vi "PDE_Fill_Setup(SubVI).vi"(6 "sample mode":i32, 8 "Error In":errorcluster, 9 "rate":dbl, 10 "number of samples":i32, 11 "Input Boolean Array":digitalwaveform[](array[waveform])) -> (0 "error out":errorcluster, 3 "Refnum out":refnum<k21>)   [LabVIEW 2018]
uses:
  <vilib>/DAQmx/write.llb/DAQmx Write (Digital 1D Wfm NChan NSamp).vi
  <vilib>/DAQmx/create/channels.llb/DAQmx Create Channel (DO-Digital Output).vi
  <vilib>/DAQmx/configure/timing.llb/DAQmx Timing (Sample Clock).vi
  <vilib>/Waveform/DWDTOps.llb/DWDT Uncompress Digital.vi
  <vilib>/DAQmx/miscellaneous.llb/DAQmx Fill In Error Info.vi
  <resource>/objmgr/daqmx.rc
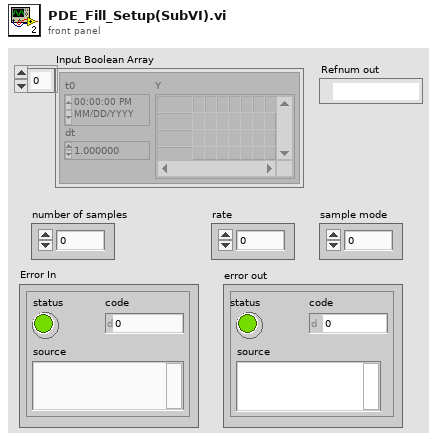
[diagram p1: front panel]
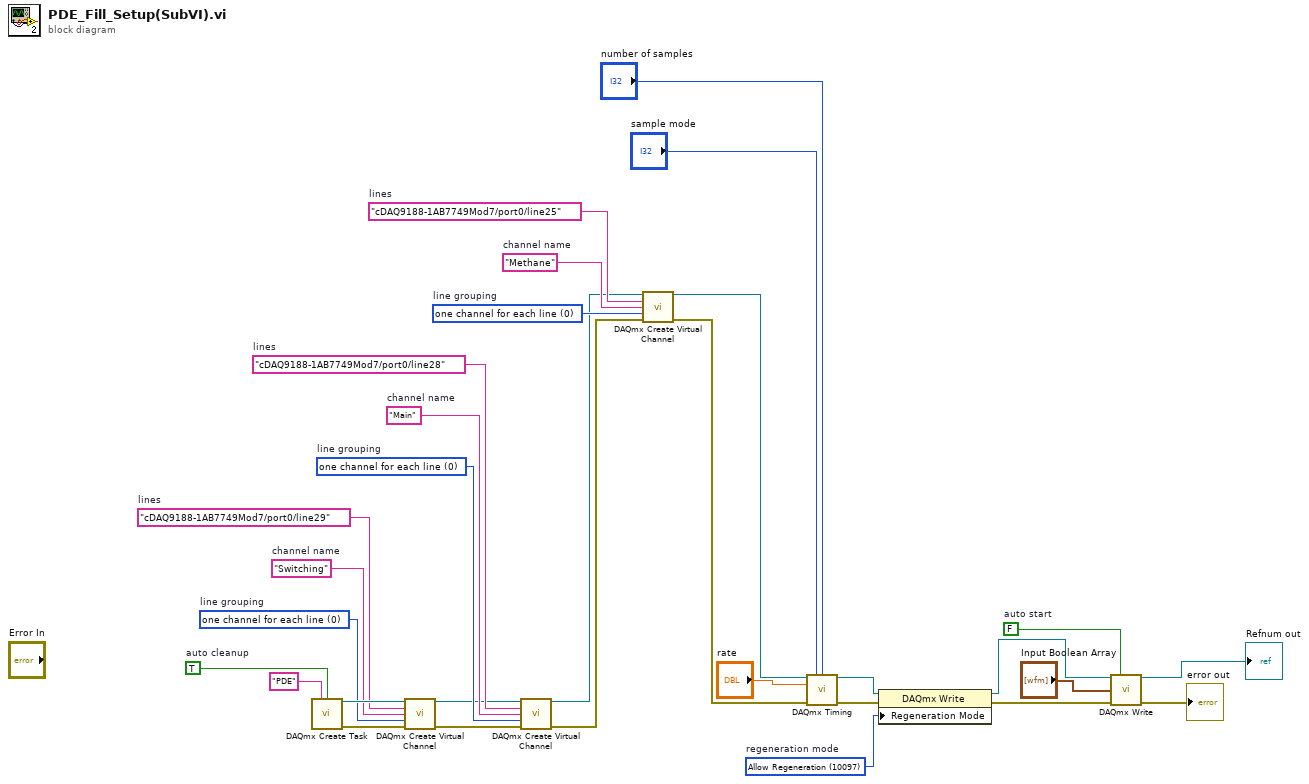
[diagram p0: block diagram]
diagram:
  w21 = 0 items=["one channel for each line", "one channel for all lines"]  # line grouping
  w22 = "Methane"  # channel name
  w20 = "cDAQ9188-1AB7749Mod7/port0/line25"  # lines
  w16 = 0 items=["one channel for each line", "one channel for all lines"]  # line grouping
  w17 = "Main"  # channel name
  w15 = "cDAQ9188-1AB7749Mod7/port0/line28"  # lines
  w11 = 0 items=["one channel for each line", "one channel for all lines"]  # line grouping
  w12 = "Switching"  # channel name
  w10 = "cDAQ9188-1AB7749Mod7/port0/line29"  # lines
  w6 = 10097 items=["Allow Regeneration"=10097, "Do Not Allow Regeneration"=10158]  # regeneration mode
  w3 = TRUE  # auto cleanup
  w1 = FALSE  # auto start
  n1 = call <vilib>:"DAQmx Create Task.vi"("new task name"="PDE", "auto cleanup"=w3) -> ("task out"=w26:refnum<k21>, "error out"=w25:errorcluster)  [unwired: 12 in]
  n2 = call-poly <vilib>:"DAQmx Create Virtual Channel.vi"("task in"=w26, "lines"=w10, "name to assign"=w12, "line grouping"=w11, "error in"=w25) -> ("task out"=w14:refnum<k21>, "error out"=w13:errorcluster)  [unwired: 9 in]
  n3 = call-poly <vilib>:"DAQmx Create Virtual Channel.vi"("task in"=w14, "lines"=w15, "name to assign"=w17, "line grouping"=w16, "error in"=w13) -> ("task out"=w19:refnum<k21>, "error out"=w18:errorcluster)  [unwired: 9 in]
  n4 = call-poly <vilib>:"DAQmx Create Virtual Channel.vi"("task in"=w19, "lines"=w20, "name to assign"=w22, "line grouping"=w21, "error in"=w18) -> ("task out"=w24:refnum<k21>, "error out"=w23:errorcluster)  [unwired: 9 in]
  n5 = call-poly <vilib>:"DAQmx Timing.vi"("task/channels in"=w24, "sample mode"="sample mode", "samples per channel"="number of samples", "rate"="rate", "error in"=w23) -> ("task out"=w5:refnum<k21>, "error out"=w4:errorcluster)  [unwired: 9 in]
  n6 = property class="DAQmx Write"(reference=w5, error in=w4, "Regeneration Mode"=w6) -> (reference out=w7:refnum<k21>, error out=w8:errorcluster)
  n7 = call-poly <vilib>:"DAQmx Write.vi"("task/channels in"=w7, "auto start"=w1, "data"="Input Boolean Array", "error in"=w8) -> ("task out"=→"Refnum out":refnum<k21>, "error out"=→"error out":errorcluster)  [unwired: 9 in, 1 out]
